vi "workspace reader.vi"() -> ()   [LabVIEW 2014]
uses:
  <vilib>/NI Veristand/Execution/Workspace/NI VeriStand - Get Single Channel Value.vi
  <vilib>/NI Veristand/Execution/Workspace/NI_VS Workspace ExecutionAPI.lvlib
panel:
  out "Value":dbl
  in  "Stop Button":bool
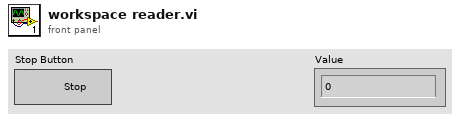
[diagram p1: front panel]
types:
  T1 = typedef "NI_VS Workspace ExecutionAPI.lvlib/WorkspaceAPI.ctl" = refnum<k24>
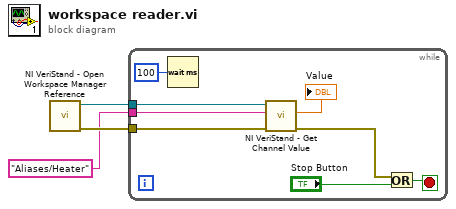
[diagram p0: block diagram]
diagram:
  n1 = call <vilib>:"NI VeriStand - Open Workspace Manager Reference.vi"() -> ("error out"=w3:errorcluster, "WorkspaceManager"=w2:T1)  [unwired: 10 in]
  n2 = while {
    tunnel: w3 -> [w11]
    tunnel: w2 -> [w10]
    tunnel: "Aliases/Heater" ("Channel") -> [w9]
    stop <- w4 stop-if-true
    n3 = Wait (ms)(milliseconds to wait=u32 100) -> ()  [unwired: 1 out]
    n4 = call-poly <vilib>:"NI VeriStand - Get Channel Value.vi"("error in (no error)"=w11, "Channel"=w9, "WorkspaceManager in"=w10) -> ("error out"=w8:errorcluster, "Value"=→"Value":dbl)  [unwired: 6 in, 1 out]
    n5 = Or(x=w8, y="Stop Button") -> (x .or. y?=w4:bool)
  }
